vi "LogLineSD.vi"(8 "error in (no error)":errorcluster, 10 "Log string":string, 11 "SerialPortRef":T1) -> (0 "error out":errorcluster, 3 "SerialPortRef 2":T1)   [LabVIEW 2016]
uses:
  <vilib>/Rock Robotics/WPI/SerialPort/WPI_SerialPortRef.ctl
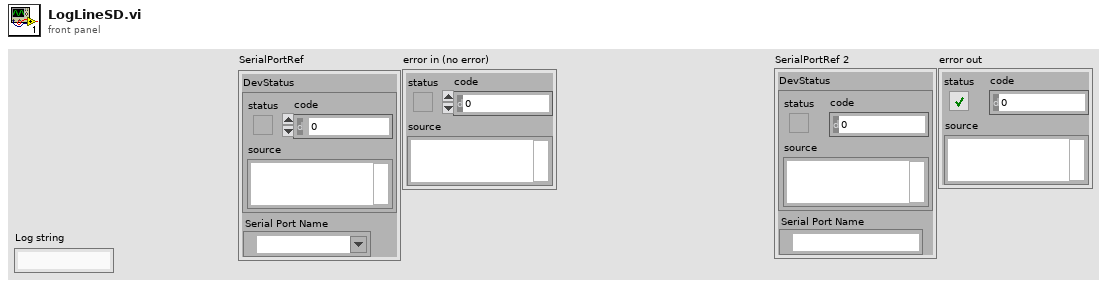
[diagram p1: front panel]
types:
  T1 = typedef "WPI_SerialPortRef.ctl" = cluster{"DevStatus":errorcluster, "Serial Port Name":refnum<visa-resource-name>}
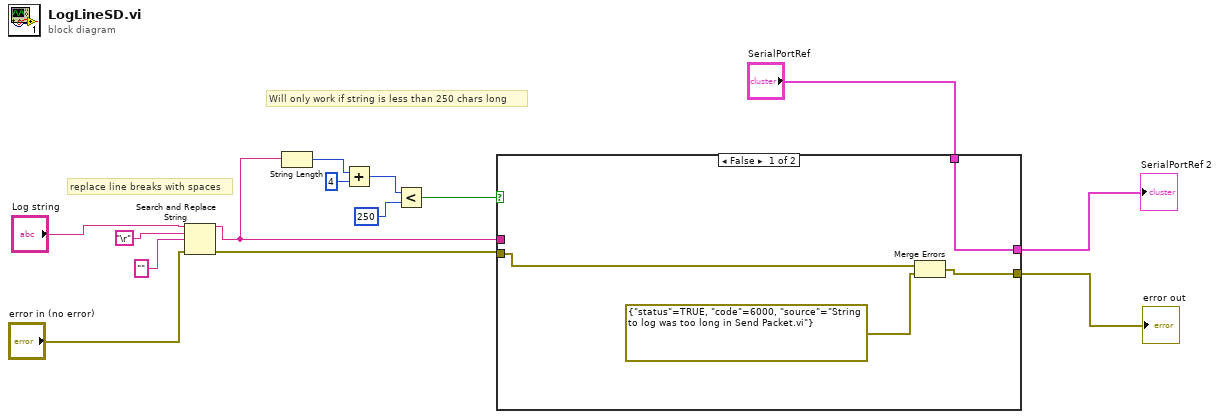
[diagram p0: block diagram]
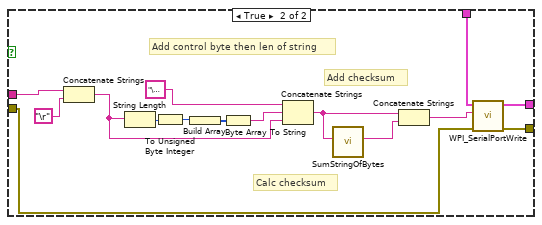
[diagram p2: hidden frame]
diagram:
  # "Will only work if string is less than 250 chars long"
  # "replace line breaks with spaces"
  n1 = Search and Replace String(input string="Log string", search string="\r", replace string="" ("replace string (\"\")"), error in="error in (no error)") -> (result string=w7:string, error out=w6:errorcluster)  [unwired: 4 in, 2 out]
  n2 = String Length(string=w7) -> (length=w9:i32)
  n3 = Add(x=w9, y=4) -> (x+y=w11:i32)
  n4 = Less?(x=w11, y=250) -> (x < y?=w8:bool)
  n5 = case shown="False" w8 {
    tunnel: w7 -> [_ w20]
    tunnel: w6 -> [w16 w19]
    tunnel: [w15 w23] -> w3
    tunnel: [w17 w22] -> w2
    tunnel: "SerialPortRef" -> [w15 w21]
    frame False {
      n6 = Merge Errors(w16, errorcluster {"status"=TRUE, "code"=6000, "source"="String to log was too long in Send Packet.vi"} ("error out")) -> (w17:errorcluster)
    }
    frame True {
      # "Add checksum"
      # "Add control byte then len of string"
      # "Calc checksum"
      n7 = Concatenate Strings(w20, "\r") -> (w26:string)
      n8 = String Length(string=w26) -> (length=w28:i32)
      n9 = To Unsigned Byte Integer(number=w28) -> (unsigned 8bit integer=w27:u8)
      n10 = Build Array(w27) -> (w33:u8[])
      n11 = Byte Array To String(unsigned byte array=w33) -> (string=w32:string)
      n12 = Concatenate Strings("\u0001", w32, w26) -> (w29:string)
      n13 = call "SumStringOfBytes.vi"("String Of Bytes"=w29) -> ("SumAsString"=w30:string)  [unwired: 10 in]
      n14 = Concatenate Strings(w29, w30) -> (w24:string)
      n15 = call <vilib>:"WPI_SerialPortWrite.vi"("error in (no error)"=w19, "Buffer"=w24, "SerialPortRef"=w21) -> ("error out"=w22:errorcluster, "SerialPortRef"=w23:T1)  [unwired: 6 in, 1 out]
    }
  }
  "SerialPortRef 2" <- w3
  "error out" <- w2
